vi "Devcon.Rescan for New Devices.vi"(8 "error in (no error)":errorcluster, 11 "DevconEXE":path=path "C:/Program Files (x86)/Windows Kits/10/Tools/x64/devcon") -> (0 "error out":errorcluster, 3 "Success":bool)   [LabVIEW 2018]
panel:
  out "StdOut":string
  out "Cmd":string
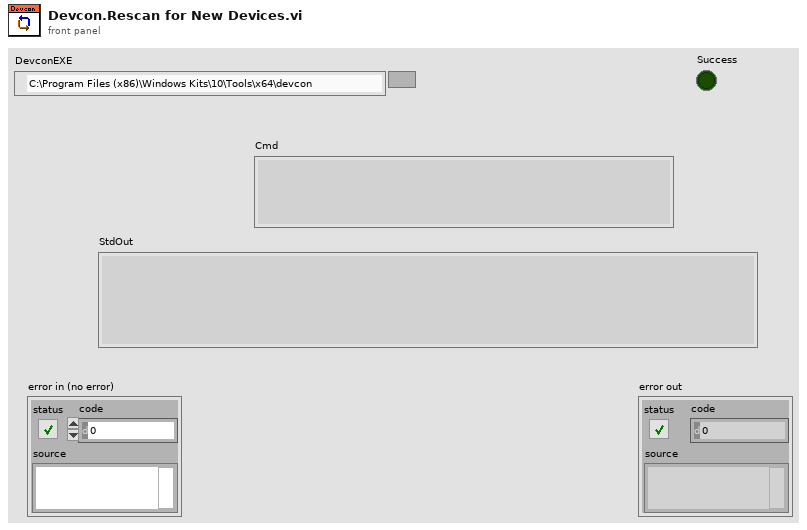
[diagram p1: front panel]
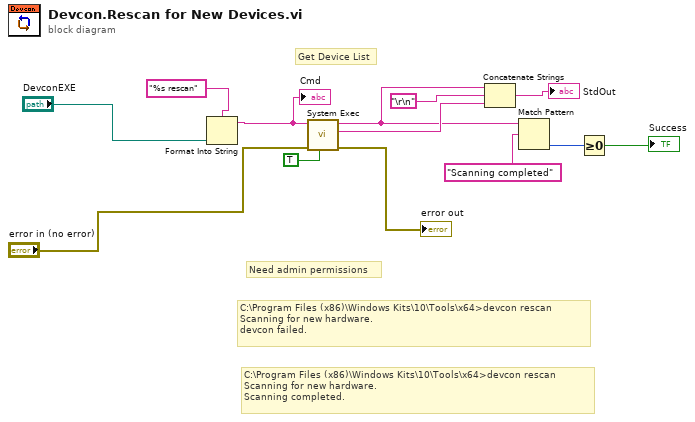
[diagram p0: block diagram]
diagram:
  # "C:\\Program Files (x86)\\Windows Kits\\10\\Tools\\x64>devcon rescan\nScanning for new hardware.\nScanning completed."
  # "Need admin permissions"
  # "C:\\Program Files (x86)\\Windows Kits\\10\\Tools\\x64>devcon rescan\nScanning for new hardware.\ndevcon failed."
  # "Get Device List"
  n1 = Format Into String(format string="%s rescan", "DevconEXE") -> (resulting string=w11:string)  [unwired: 2 in, 1 out]
  "Cmd" <- w11
  n2 = call <vilib>:"System Exec.vi"("run minimized? (F)"=TRUE, "error in (no error)"="error in (no error)", "command line"=w11) -> ("error out"=→"error out":errorcluster, "standard error"=w4:string, "standard output"=w3:string)  [unwired: 5 in, 1 out]
  n3 = Concatenate Strings(w3, "\r\n", w4) -> (→"StdOut":string)
  n4 = Match Pattern(string=w3, regular expression="Scanning completed") -> (offset past match=w6:i32)  [unwired: 1 in, 3 out]
  n5 = Greater Or Equal To 0?(x=w6) -> (x >= 0?=→"Success":bool)
